vi "dispose dataset.vi"(8 "error in":errorcluster, 11 "basic HTTP handler dataset in":refnum<class "basic HTTP handler dataset.lvclass">) -> (0 "error out":errorcluster)   [LabVIEW 2016, in "basic HTTP handler dataset.lvclass"]
uses:
  basic HTTP handler dataset.lvclass
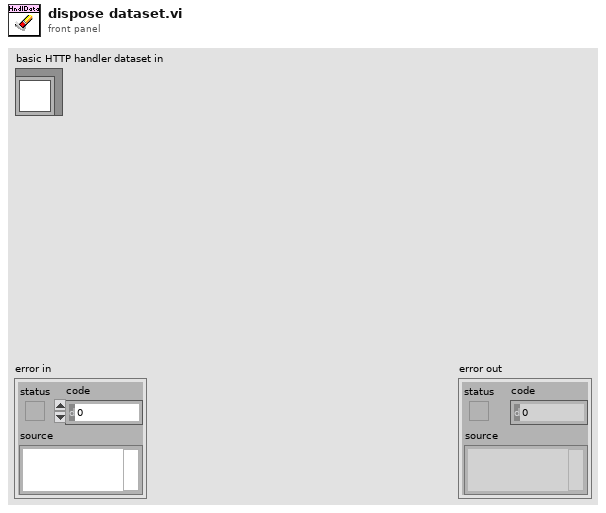
[diagram p1: front panel]
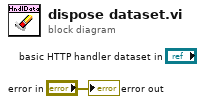
[diagram p0: block diagram]
diagram:
  "error out" <- "error in"
